vi "RT Communications Loop.vi"(9 "Comms data":T1={"Parameters"={"error writer name"="error writer", "command reader name"="command reader", "error buffer size"=16, "command buffer size"=16, "scanivalveIP"="", "scanivalvePeriod"=16}, "Variables"={"listen schedule"=0, "incident buffer"=[], "command stream"="", "error stream"="", "waiting for command stream connect"=FALSE, "waiting for error stream connect"=FALSE, "scanivalve connection"=refnum, "scanivalveScheduleID"=16}}, 11 "RT Queues":T3) -> ()   [LabVIEW 2018]
uses:
  Type Defs/Queues cluster.ctl
  Chris VIs/Message Scheduler/message scheduler.lvclass
  Communications loop/comms data.ctl
  Type Defs/generic incident.ctl
  Turbo Group LabVIEW repository/Main Controller SVE/Controller Data/Cabinet data FGV states.ctl
  Chris VIs/Message Scheduler/generic message queue/standard message queue/standard message.lvclass
  \\Mac\Home/OneDrive - Imperial College London/LabVIEW/Chris VIs/Message Scheduler/generic message queue/generic message.lvclass
  Queue VIs/De-queue RT comms element.vi
  Scanivalve API project/polymorphic vis/read scanivalve data.vi
  Queue VIs/En-queue RT data element.vi
  Queue VIs/Close RT comms queue.vi
  Chris VIs/Message Scheduler/scheduled message/scheduled message.lvclass
  Turbo Group LabVIEW repository/Main Controller SVE/Lab123H main cabinet API.lvlib
  Queue VIs/En-queue RT comms element.vi
panel:
  out "buffered messages":i32
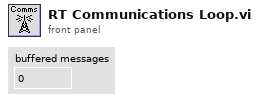
[diagram p1: front panel]
types:
  T1 = typedef "comms data.ctl" = cluster{"Parameters":cluster{"error writer name":string, "command reader name":string, "error buffer size":i32, "command buffer size":i32, "scanivalveIP":string, "scanivalvePeriod":u16}, "Variables":cluster{"listen schedule":u32, "incident buffer":T2[], "command stream":refnum<k21>, "error stream":refnum<k21>, "waiting for command stream connect":bool, "waiting for error stream connect":bool, "scanivalve connection":refnum<k5>, "scanivalveScheduleID":u32}}
  T2 = typedef "generic incident.ctl" = cluster{"timestamp":timestamp, "type":string, "Variant":variant}
  T3 = typedef "Queues cluster.ctl" = cluster{"RT Message":refnum<queue>, "RT Comms":refnum<queue>, "RT Data":refnum<queue>, "RT FIFO":refnum<queue>, "message scheduler":refnum<class "message scheduler.lvclass">}
  T4 = typedef "Cabinet data FGV states.ctl" = enum16{"connect", "read", "disconnect"}
  T5 = typedef "MainCabinetDataRead.ctl" = cluster{"CurrentIn":cluster{"MainValveFeed(%)":sgl, "SecValveFeed(%)":sgl, "AirMassFlow(Kg/s)":sgl, "StatorOilPressure(BarG)":sgl, "BearingOilPressure(BarG)":sgl}, "VoltageIn":cluster{"AmbientPressure(Pa)":sgl}, "Indicators":cluster{"AirMassFlowOK":bool, "EMstopOK":bool, "Thermocouple Error":bool, "MainCabinet_CPU (%)":dbl, "Error":bool}, "Temperature":cluster{"LabTemp":dbl, "HeaterTemp":dbl, "Oil TC 1":dbl, "Oil TC 2":dbl, "Oil TC 3":dbl, "Oil TC 4":dbl, "Oil TC 5":dbl, "Oil TC 6":dbl}, "Flowrates (L/min)":cluster{"BearingOil":dbl, "StatorOil":dbl, "BearingFlow":bool, "StatorFlow":bool}}
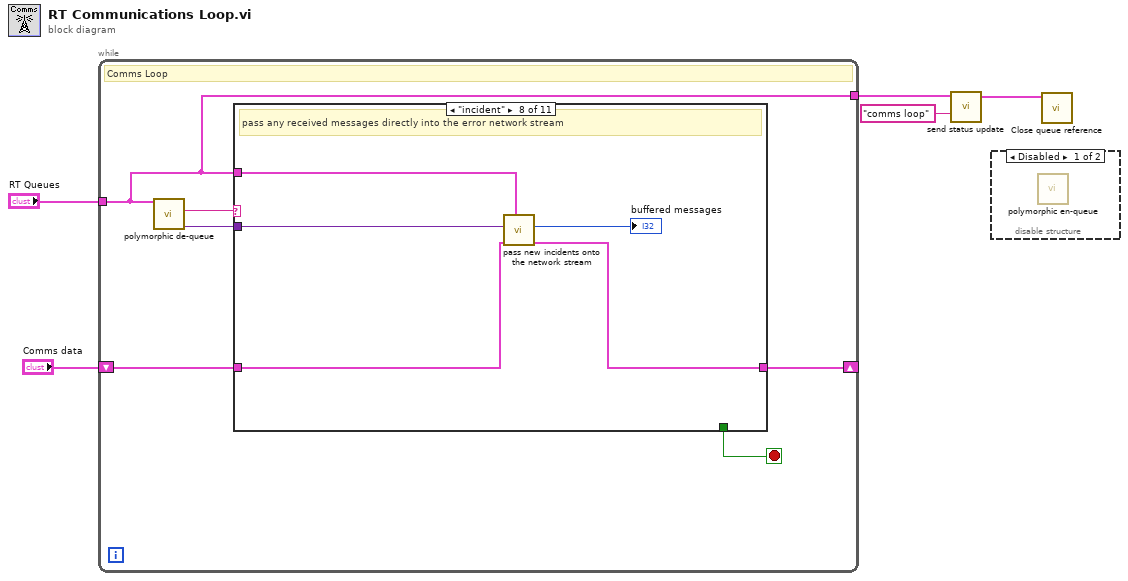
[diagram p0: block diagram]
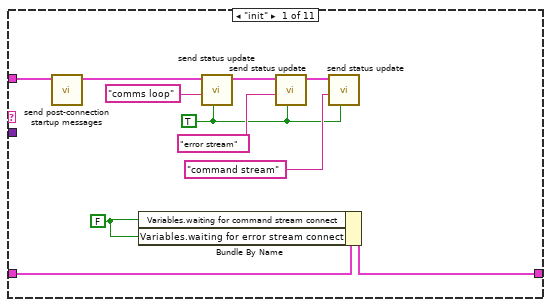
[diagram p3: hidden frame]
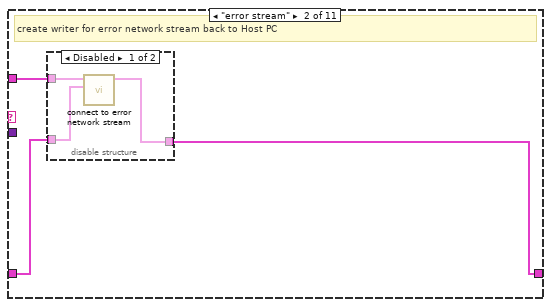
[diagram p4: hidden frame]
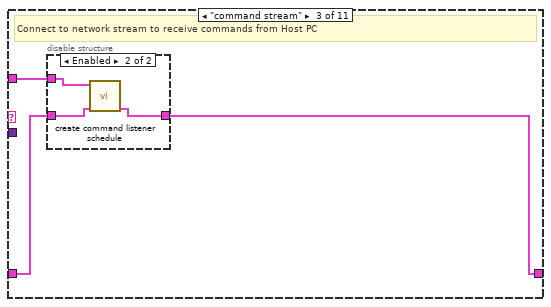
[diagram p6: hidden frame]
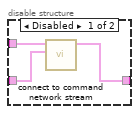
[diagram p7: hidden frame]
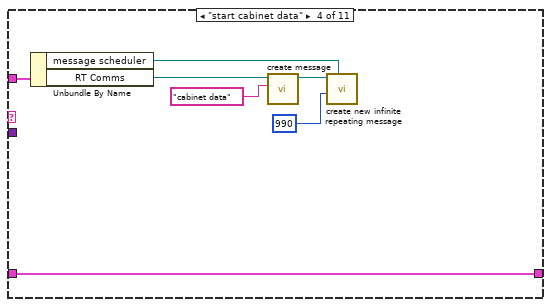
[diagram p8: hidden frame]
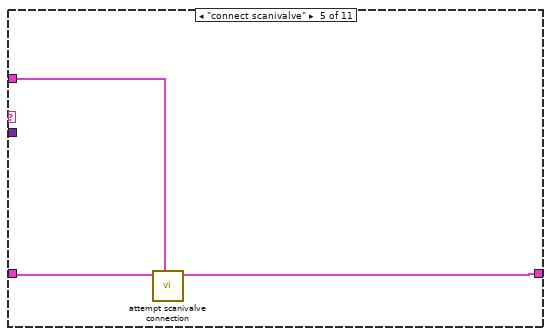
[diagram p9: hidden frame]
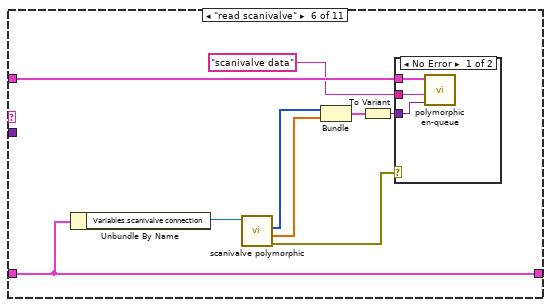
[diagram p10: hidden frame]
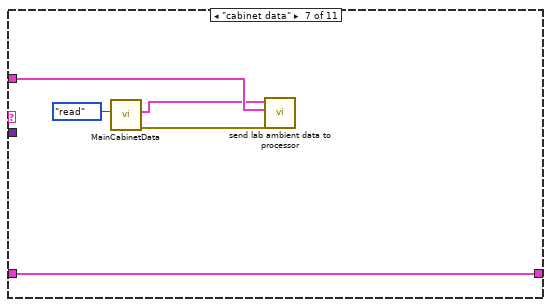
[diagram p12: hidden frame]
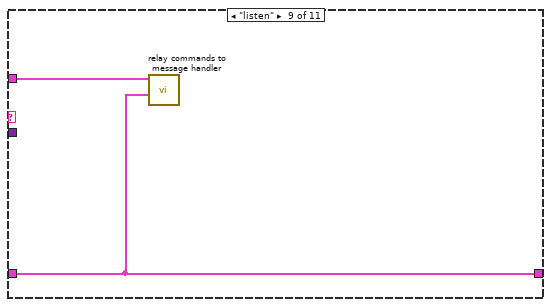
[diagram p13: hidden frame]
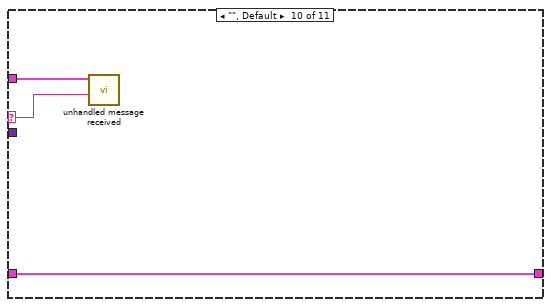
[diagram p14: hidden frame]
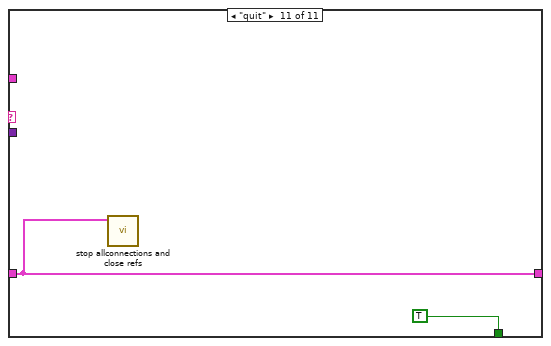
[diagram p15: hidden frame]
diagram:
  n1 = while {
    tunnel: "RT Queues" -> [w6]
    tunnel: [w6] -> w3
    shift-right: [w7] -> _
    shift-left: "Comms data" -> [w8]
    stop <- w9 stop-if-true
    # "Comms Loop"
    n2 = call-poly "polymorphic de-queue.vi"("RT Queues"=w6) -> ("Data"=w10:variant, "Message"=w11:string)  [unwired: 8 in, 1 out]
    n3 = case shown="\"incident\"" w11 {
      selector: w11 -> [_ _ _ _ _ _ _ _ _ w73 _]
      tunnel: w10 -> [_ _ _ _ _ _ _ w70 _ _ _]
      tunnel: [_ _ _ _ _ _ _ _ _ _ TRUE] -> w9
      tunnel: w6 -> [w22 w23 w30 w41 w46 w55 w64 w66 w72 w74 _]
      tunnel: w8 -> [w21 w25 w32 w45 w47 w57 w65 w69 w71 w75 w76]
      tunnel: [w19 w24 w31 w45 w48 w57 w65 w68 w71 w75 w76] -> w7
      frame "init" {
        w18 = FALSE ("Variables.waiting for command stream connect")
        w12 = TRUE
        n4 = call "send post-connection startup messages.vi"("RT Queues"=w22) -> ("RT Queues out"=w17:T3)  [unwired: 10 in]
        n5 = Bundle By Name(cluster=w21, "Variables.waiting for command stream connect"=w18, "Variables.waiting for error stream connect"=w18) -> (w19:T1)
        n6 = call "send status update.vi"("status (F)"=w12, "subject"="comms loop" ("Message"), "RT Queues"=w17) -> ("RT Queues out"=w13:T3)  [unwired: 8 in]
        n7 = call "send status update.vi"("status (F)"=w12, "subject"="error stream" ("Message"), "RT Queues"=w13) -> ("RT Queues out"=w15:T3)  [unwired: 8 in]
        n8 = call "send status update.vi"("status (F)"=w12, "subject"="command stream" ("Message"), "RT Queues"=w15) -> ()  [unwired: 8 in, 1 out]
      }
      frame "error stream" {
        # "create writer for error network stream back to Host PC"
        n9 = disable-structure shown="Disabled" {
          disable-tunnel: w25 -> [w28 w29]
          disable-tunnel: [w27 w29] -> w24
          disable-tunnel: w23 -> [w26 _]
          frame Disabled {
            n10 = call "connect to error network stream.vi"("Comms data in"=w28, "RT Queues"=w26) -> ("Comms data out"=w27:T1)  [unwired: 9 in]
          }
          frame Enabled {
          }
        }
      }
      frame "command stream" {
        # "Connect to network stream to receive commands from Host PC"
        n11 = disable-structure shown="Enabled" {
          disable-tunnel: w32 -> [w35 w37]
          disable-tunnel: [w34 w36] -> w31
          disable-tunnel: w30 -> [w33 w38]
          frame Disabled {
            n12 = call "connect to command network stream.vi"("Comms data in"=w35, "RT Queues"=w33) -> ("Comms data out"=w34:T1)  [unwired: 9 in]
          }
          frame Enabled {
            n13 = call "create command listener schedule.vi"("Comms data in"=w37, "RT Queues"=w38) -> ("Comms data out"=w36:T1)  [unwired: 9 in]
          }
        }
      }
      frame "start cabinet data" {
        n14 = Unbundle By Name(w41) -> ("message scheduler"=w39:refnum<class "message scheduler.lvclass">, "RT Comms"=w40:refnum<queue>)
        n15 = call "create message.vi"("message"="cabinet data", "queue ref"=w40) -> ("standard message out"=w43:refnum<class "standard message.lvclass">)  [unwired: 8 in, 1 out]
        n16 = call "create new infinite repeating message.vi"("message scheduler"=w39, "ms delay"=u32 990, "message"=w43) -> ()  [unwired: 7 in, 2 out]
      }
      frame "connect scanivalve" {
        n17 = call "attempt scanivalve connection.vi"("RT Queues"=w46, "Comms data in"=w47) -> ("Comms data out"=w48:T1)  [unwired: 9 in]
      }
      frame "read scanivalve" {
        n18 = Unbundle By Name(w57) -> ("Variables.scanivalve connection"=w56:refnum<k5>)
        n19 = call-poly "scanivalve polymorphic.vi"("scanivalve connection in"=w56) -> ("error out"=w53:errorcluster, "allPressures"=w52:dbl[], "Ports"=w49:i32[])  [unwired: 7 in, 1 out]
        n20 = Bundle("Ports"=w49, "allPressures"=w52) -> (w50:cluster{"Ports":i32[], "allPressures":dbl[]})  [unwired: 1 in]
        n21 = To Variant(anything=w50) -> (Variant=w51:variant)
        n22 = case shown="No Error" w53 {
          tunnel: w55 -> [w60 _]
          tunnel: "scanivalve data" ("Message") -> [w59 _]
          tunnel: w51 -> [w58 _]
          frame No Error {
            n23 = call-poly "polymorphic en-queue.vi"("Data"=w58, "Message"=w59, "RT Queues"=w60) -> ()  [unwired: 6 in, 3 out]
          }
          frame Error {
          }
        }
      }
      frame "cabinet data" {
        n24 = call "MainCabinetData.vi"("Action"=Cabinet_data_FGV_states."read") -> ("error IO"=w61:errorcluster, "read data"=w63:T5)  [unwired: 8 in, 1 out]
        n25 = call "send lab ambient data to processor.vi"("error in (no error)"=w61, "RT Queues"=w64, "read data"=w63) -> ()  [unwired: 9 in]
      }
      frame "incident" {
        # "pass any received messages directly into the error network stream"
        n26 = call "pass new incidents onto the network stream.vi"("RT Queues"=w66, "Comms data"=w69, "incident"=w70) -> ("Comms data out"=w68:T1, "buffered messages"=→"buffered messages":i32)  [unwired: 7 in]
      }
      frame "listen" {
        n27 = call "relay commands to message handler.vi"("Comms data"=w71, "RT Queues"=w72) -> ()  [unwired: 10 in]
      }
      frame "", Default {
        n28 = call "unhandled message received.vi"("unhandled message"=w73, "RT Queues"=w74) -> ()  [unwired: 10 in]
      }
      frame "quit" {
        n29 = call "stop allconnections and close refs.vi"("Comms data"=w76) -> ()  [unwired: 11 in]
      }
    }
  }
  n30 = call "send status update.vi"("subject"="comms loop" ("Message"), "RT Queues"=w3) -> ("RT Queues out"=w2:T3)  [unwired: 9 in]
  n31 = disable-structure shown="Disabled" {
    frame Disabled {
      n32 = call-poly "polymorphic en-queue.vi"() -> ()  [unwired: 11 in, 1 out]
    }
    frame Enabled {
    }
  }
  n33 = call-poly "Close queue reference.vi"("RT Queues"=w2) -> ()  [unwired: 11 in]
